vi "PresetFire.vi"   [LabVIEW 2015]
uses:
  <vilib>/Rock Robotics/Network Tables/NT Read Number.vi
types:
  T1 = typedef "WPI_ServoDeviceRef.ctl" = cluster{"DeviceStatus":errorcluster, "PWM Channel":T2, "DeadBand":T3}
  T2 = typedef "FPGA_DIOPWMChannel.ctl" = enum8{"PWM 0", "PWM 1", "PWM 2", "PWM 3", "PWM 4", "PWM 5", "PWM 6", "PWM 7", "PWM 8", "PWM 9", "PWM MXP 0", "PWM MXP 1", "PWM MXP 2", "PWM MXP 3", "PWM MXP 4", "PWM MXP 5", "PWM MXP 6", "PWM MXP 7", "PWM MXP 8", "PWM MXP 9", "Invalid"}
  T3 = typedef "WPI_PWMDeadband.ctl" = cluster{"Name":string, "maxPositivePwm":i32, "minPositivePwm":i32, "centerPwm":i32, "maxNegativePwm":i32, "minNegativePwm":i32, "angularRange":u16}
  T4 = typedef "WPI_MotorControlDeviceRef.ctl" = cluster{"DeviceStatus":errorcluster, "Type":T5, "PWM":cluster{"PWM Channel":T2, "DeadBand":T3}, "CAN":cluster{"Device Number":u8, "Control Mode":T6, "Semaphore":T7, "Max Vout":dbl, "TalonSRX Control Mode":T8}, "Invert":bool}
  T5 = typedef "WPI_MotorControlType.ctl" = enum16{"PWM", "CAN", "CANTalonSRX"}
  T6 = typedef "WPI_CANJaguar_ControlMode.ctl" = enum8{"Percent VBus", "Current", "Speed", "Position", "Voltage"}
  T7 = typedef "Semaphore RefNum" = refnum<k1>
  T8 = typedef "WPI_CANTalonSRX_APIControlMode.ctl" = enum8{"Percent VBus", "Speed", "Position", "Slave", "Unchanged / Invalid", "Voltage Compensation", "Current", "Motion Profile"}
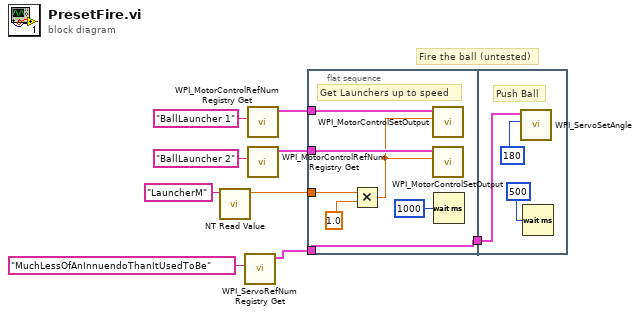
[diagram p0: block diagram]
diagram:
  # "Fire the ball (untested)"
  n1 = call-poly <vilib>:"NT Read Value.vi"("Name"="LauncherM") -> ("Numeric"=w4:dbl)  [unwired: 9 in, 1 out]
  n2 = call <vilib>:"WPI_ServoRefNum Registry Get.vi"("refnum name"="MuchLessOfAnInnuendoThanItUsedToBe") -> ("ServoDeviceRef"=w3:T1)  [unwired: 9 in, 1 out]
  n3 = call <vilib>:"WPI_MotorControlRefNum Registry Get.vi"("refnum name"="BallLauncher 1") -> ("MotorControlDevRef"=w7:T4)  [unwired: 9 in, 1 out]
  n4 = call <vilib>:"WPI_MotorControlRefNum Registry Get.vi"("refnum name"="BallLauncher 2") -> ("MotorControlDevRef"=w6:T4)  [unwired: 9 in, 1 out]
  n5 = flat-sequence {
    tunnel: w7 -> [w16]
    tunnel: w6 -> [w15]
    tunnel: w4 -> [w13]
    tunnel: w3 -> [w10]
    tunnel: [w10] -> w2
    tunnel: w2 -> [w18]
    frame #0 {
      # "Get Launchers up to speed"
      n6 = Multiply(x=w13, y=1.0 ("x")) -> (x*y=w14:dbl)
      n7 = call <vilib>:"WPI_MotorControlSetOutput.vi"("Output"=w14, "MotorControlDevRef"=w16) -> ()  [unwired: 7 in, 3 out]
      n8 = call <vilib>:"WPI_MotorControlSetOutput.vi"("Output"=w14, "MotorControlDevRef"=w15) -> ()  [unwired: 7 in, 3 out]
      n9 = Wait (ms)(milliseconds to wait=u32 1000) -> ()  [unwired: 1 out]
    }
    frame #1 {
      # "Push Ball"
      n10 = call <vilib>:"WPI_ServoSetAngle.vi"("Angle"=180, "ServoDeviceRef"=w18) -> ()  [unwired: 8 in, 2 out]
      n11 = Wait (ms)(milliseconds to wait=u32 500) -> ()  [unwired: 1 out]
    }
  }
